vi "clearTCPBuffer.vi"(9 "data in":string, 11 "connection ID":refnum<k5>) -> (1 "data out":string, 3 "connection ID out":refnum<k5>)   [LabVIEW 2020]
panel:
  out "data out 3":string
  in  "error in":errorcluster
  out "bytes to read":i32
  out "data out 2":string
  out "Numeric":i32
  out "error IO":errorcluster
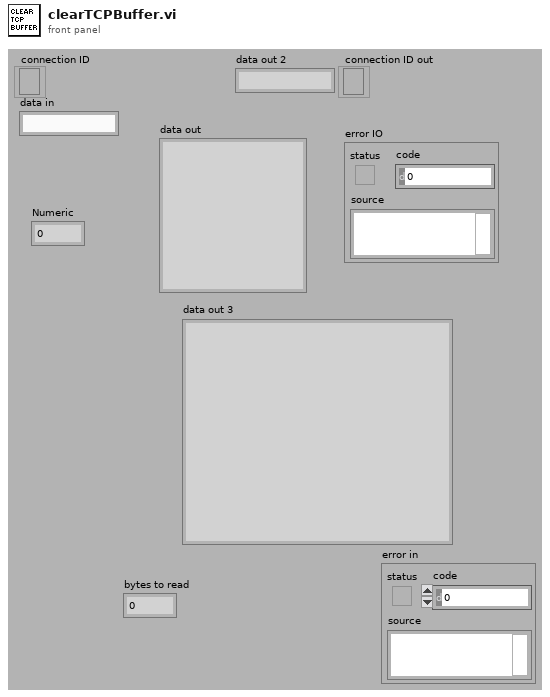
[diagram p1: front panel]
types:
  T1 = enum16{"Standard", "Buffered", "CRLF", "Immediate"}
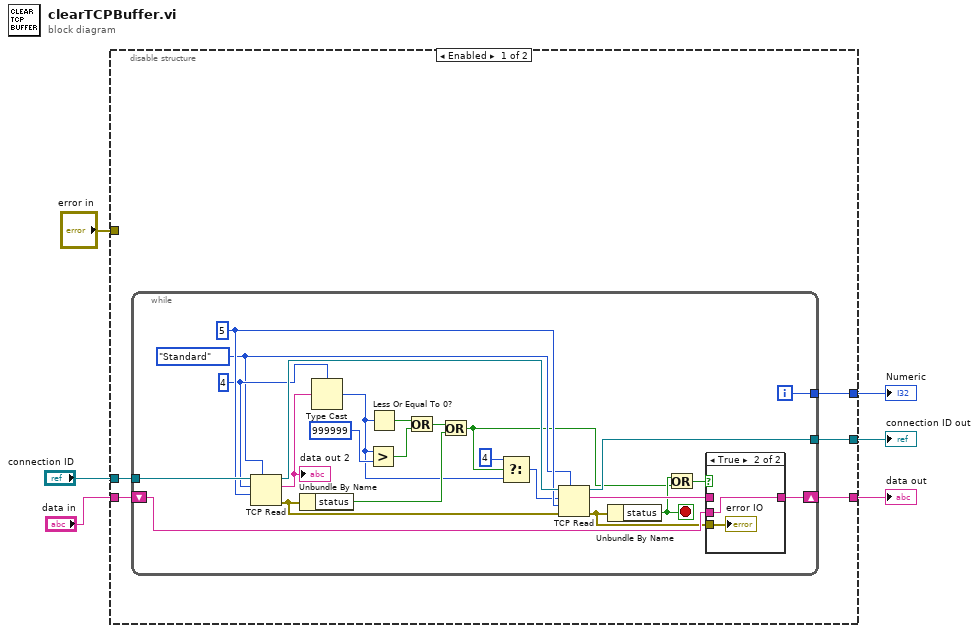
[diagram p0: block diagram]
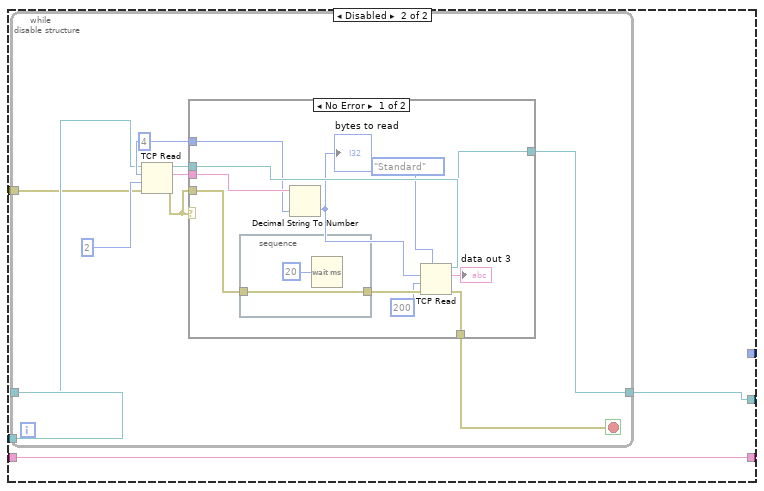
[diagram p3: hidden frame]
diagram:
  n1 = disable-structure shown="Enabled" {
    disable-tunnel: "connection ID" -> [w11 w41]
    disable-tunnel: [w10 w40] -> w5
    disable-tunnel: "data in" -> [w9 w42]
    disable-tunnel: [w8 w42] -> w3
    disable-tunnel: [w7 _] -> w2
    disable-tunnel: "error in" -> [_ w39]
    frame Enabled {
      n2 = while {
        tunnel: w11 -> [w34]
        tunnel: [w33] -> w10
        shift-right: [w31] -> w8
        shift-left: w9 -> [w30]
        tunnel: [w29] -> w7
        i -> [w29]
        stop <- w15 stop-if-true
        w16 = T1."Standard" ("mode (standard)")
        w32 = 5 ("timeout ms (25000)")
        w27 = 4
        n3 = TCP Read(connection ID=w34, bytes to read=w27, 7:w16, 9:w32) -> (connection ID out=w35:refnum<k5>, data out=w28:string, error out=w23:errorcluster)  [unwired: 1 in]
        "data out 2" <- w28
        n4 = Unbundle By Name(w23) -> ("status"=w21:bool)
        n5 = Type Cast(type=w27, x=w28) -> (*(type *) &x=w19:i32)
        n6 = Greater?(x=w19, y=999999) -> (0:w24:bool)
        n7 = Less Or Equal To 0?(x=w19) -> (x <= 0?=w25:bool)
        n8 = Or(x=w25, y=w24) -> (x .or. y?=w22:bool)
        n9 = Or(x=w22, y=w21) -> (x .or. y?=w14:bool)
        n10 = Select(t=4, s=w14, f=w19) -> (s? t:f=w17:i32)
        n11 = TCP Read(connection ID=w35, bytes to read=w17, error in (no error)=w23, 7:w16, 9:w32) -> (connection ID out=w33:refnum<k5>, data out=w20:string, error out=w12:errorcluster)
        n12 = Unbundle By Name(w12) -> ("status"=w15:bool)
        n13 = Or(x=w15, y=w14) -> (x .or. y?=w13:bool)
        n14 = case shown="True" w13 {
          tunnel: [w36 w38] -> w31
          tunnel: w20 -> [w36 _]
          tunnel: w30 -> [_ w38]
          tunnel: w12 -> [_ w37]
          frame False {
          }
          frame True {
            "error IO" <- w37
          }
        }
      }
    }
    frame Disabled {
      n15 = while {
        tunnel: w41 -> [w47]
        tunnel: [w46] -> w40
        tunnel: w39 -> [w44]
        stop <- w45 stop-if-true
        w49 = 4 ("bytes to read")
        n16 = TCP Read(connection ID=w47, bytes to read=w49, error in (no error)=w44, 9:2 ("timeout ms (25000)")) -> (connection ID out=w50:refnum<k5>, data out=w51:string, error out=w43:errorcluster)  [unwired: 1 in]
        n17 = case shown="No Error" w43 {
          tunnel: w43 -> [w61 w66]
          tunnel: w51 -> [w60 _]
          tunnel: w50 -> [w59 w65]
          tunnel: w49 -> [w58 _]
          tunnel: [w55 w65] -> w46
          tunnel: [w54 w66] -> w45
          frame No Error {
            n18 = stacked-sequence {
              tunnel: w61 -> [w63]
              tunnel: [w63] -> w62
              frame #0 {
                n19 = Wait (ms)(milliseconds to wait=u32 20) -> ()  [unwired: 1 out]
              }
            }
            n20 = Decimal String To Number(string=w60, default (0L)=w58) -> (number=w56:i32)  [unwired: 1 in, 1 out]
            "bytes to read" <- w56
            n21 = TCP Read(connection ID=w59, bytes to read=w56, error in (no error)=w62, 7:T1."Standard" ("mode (standard)"), 9:200 ("timeout ms (25000)")) -> (connection ID out=w55:refnum<k5>, data out=→"data out 3":string, error out=w54:errorcluster)
          }
          frame Error {
          }
        }
      }
    }
  }
  "connection ID out" <- w5
  "data out" <- w3
  "Numeric" <- w2
